vi "SplitTransferAndReceive.vi"(8 "error in":errorcluster caption="错误输入（无错误）", 11 "StrArrayIn":string[][](array[string])) -> (0 "error out":errorcluster caption="错误输出", 1 "Receive":string[][](array[string]), 3 "Transfer":string[][](array[string]))   [LabVIEW 2013]
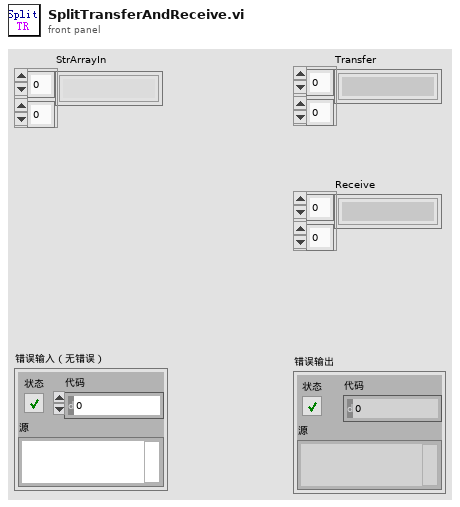
[diagram p1: front panel]
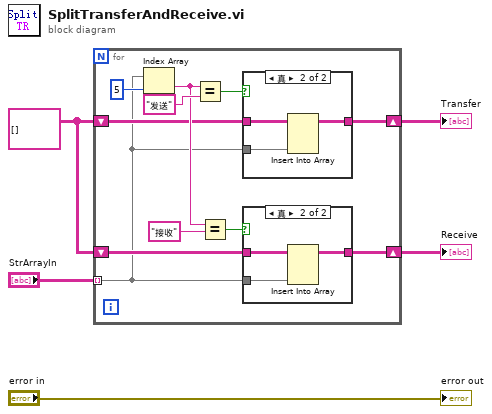
[diagram p0: block diagram]
diagram:
  w4 = string[][] []
  n1 = for {
    tunnel: "StrArrayIn" -> [w6] mode=indexing
    shift-right: [w10] -> w2
    shift-left: w4 -> [w11]
    shift-right: [w7] -> w1
    shift-left: w4 -> [w8]
    n2 = Index Array(array=w6, index=5 ("索引")) -> (element=w13:string)
    n3 = Equal?(x=w13, y="发送") -> (x = y?=w14:bool)
    n4 = Equal?(x=w13, y="接收") -> (x = y?=w9:bool)
    n5 = case shown="真" w14 {
      tunnel: w11 -> [w21 w24]
      tunnel: [w21 w23] -> w10
      tunnel: w6 -> [_ w22]
      frame False {
      }
      frame True {
        n6 = Insert Into Array(array=w24, new element=w22) -> (w23:string[][])  [unwired: 2 in]
      }
    }
    n7 = case shown="真" w9 {
      tunnel: w8 -> [w17 w20]
      tunnel: [w17 w19] -> w7
      tunnel: w6 -> [_ w18]
      frame False {
      }
      frame True {
        n8 = Insert Into Array(array=w20, new element=w18) -> (w19:string[][])  [unwired: 2 in]
      }
    }
  }
  "Transfer" <- w2
  "Receive" <- w1
  "error out" <- "error in"
